vi "test_connection_SampleHandler.vi"(8 "error in (no error)":errorcluster caption="エラー入力（エラーなし）", 11 "VISAリソース名":refnum<visa-resource-name>) -> (0 "error out":errorcluster caption="エラー出力", 1 "Motor count":i32, 2 "connected?":bool, 3 "VISAリソース名（出力）":refnum<visa-resource-name>)   [LabVIEW 2017]
uses:
  <vilib>/Instr/_visa.llb/VISA Configure Serial Port (Instr).vi
panel:
  out "レスポンス":string
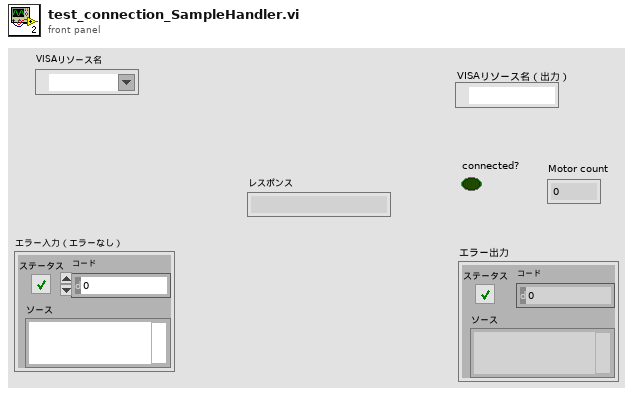
[diagram p1: front panel]
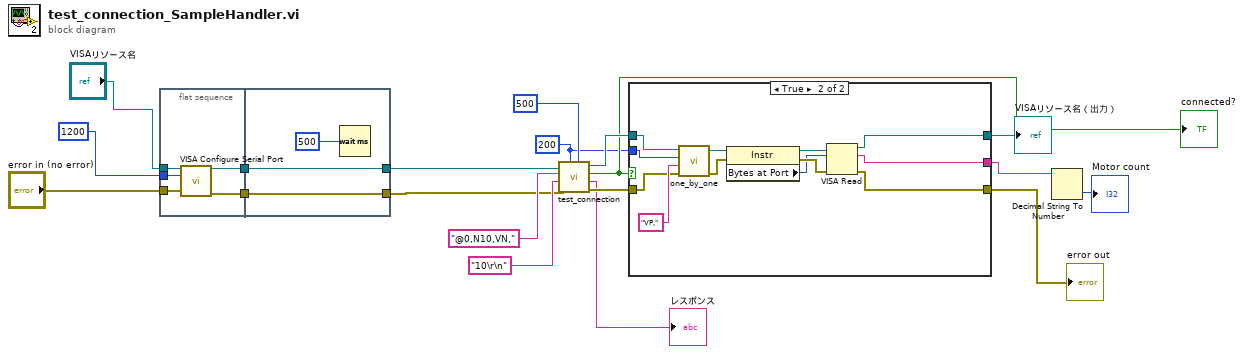
[diagram p0: block diagram]
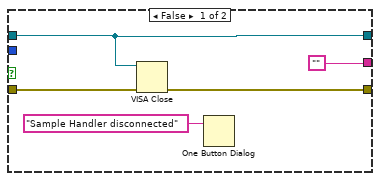
[diagram p2: hidden frame]
diagram:
  w3 = 200
  n1 = flat-sequence {
    tunnel: "VISAリソース名" -> [w24]
    tunnel: "error in (no error)" -> [w23]
    tunnel: 1200 -> [w22]
    tunnel: [w21] -> w7
    tunnel: [w20] -> w6
    tunnel: [w26] -> w8
    tunnel: [w27] -> w9
    tunnel: w7 -> [w27]
    tunnel: w6 -> [w26]
    frame #0 {
      n2 = call-poly "VISA Configure Serial Port"("VISA resource name"=w24, "baud rate (9600)"=w22, "error in (no error)"=w23) -> ("VISA resource name out"=w21:refnum<visa-resource-name>, "error out"=w20:errorcluster)  [unwired: 11 in]
    }
    frame #1 {
      n3 = Wait (ms)(milliseconds to wait=500) -> ()  [unwired: 1 out]
    }
  }
  n4 = call "test_connection.vi"("読み取り前待機 (500 ms)"=500, "文字送信間隔 (500 ms)"=w3, "error in (no error)"=w8, "想定レスポンス"="10\r\n", "コマンド"="@0,N10,VN,", "VISAリソース名"=w9) -> ("error out"=w17:errorcluster, "レスポンス"=→"レスポンス":string, "一致？"=w14:bool, "VISAリソース名 （出力）"=w16:refnum<visa-resource-name>)  [unwired: 2 in]
  "connected?" <- w14
  n5 = case shown="TRUE" w14 {
    tunnel: w17 -> [w32 w41]
    tunnel: w16 -> [w29 w44]
    tunnel: [w30 w34] -> w15
    tunnel: [w29 w35] -> w10
    tunnel: w3 -> [_ w43]
    tunnel: ["" w33] -> w1
    frame False {
      n6 = VISA Close(VISA resource name=w29, error in (no error)=w32) -> (error out=w30:errorcluster)
      n7 = One Button Dialog(message="Sample Handler disconnected") -> ()  [unwired: 1 in, 1 out]
    }
    frame True {
      n8 = call "one_by_one.vi"("error in (no error)"=w41, "入力文字"="VP,", "待機 (200ms)"=w43, "VISAリソース名"=w44) -> ("error out"=w39:errorcluster, "VISAリソース名出力"=w40:refnum<visa-resource-name>)  [unwired: 6 in]
      n9 = property class="Instr"(reference=w40, error in=w39) -> (reference out=w37:refnum<visa-resource-name>, error out=w38:errorcluster, "Bytes at Port"=w36:u32)
      n10 = VISA Read(VISA resource name=w37, byte count=w36, error in (no error)=w38) -> (VISA resource name out=w35:refnum<visa-resource-name>, read buffer=w33:string, error out=w34:errorcluster)  [unwired: 1 out]
    }
  }
  "error out" <- w15
  "VISAリソース名（出力）" <- w10
  n11 = Decimal String To Number(string=w1) -> (number=→"Motor count":i32)  [unwired: 2 in, 1 out]
